vi "Example UDP send MC commands loop.vi"() -> ()   [LabVIEW 2009]
uses:
  UDP Lib/UDP Network Location.ctl
  Remote Control/Motor Command.ctl
  Remote Control/Message Type.ctl
panel:
  in  "Destination Location":T1
  in  "stop":bool
  in  "Turn":i16
  in  "Speed":i16
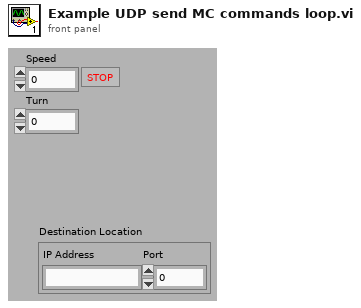
[diagram p1: front panel]
types:
  T1 = typedef "UDP Network Location.ctl" = cluster{"IP Address":string, "Port":u16}
  T2 = typedef "UDP Base.ctl" = cluster{"UDP Session":refnum<k16>, "UDP Socket Params":T3}
  T3 = typedef "UDP Socket Params.ctl" = cluster{"Local Port":u16, "Read Timeout":i32, "Write Timeout":i32}
  T4 = typedef "Message Type.ctl" = enum16{"Motor Command", "Debug Data"}
  T5 = typedef "Motor Command.ctl" = cluster{"Speed":i16, "Turn":i16}
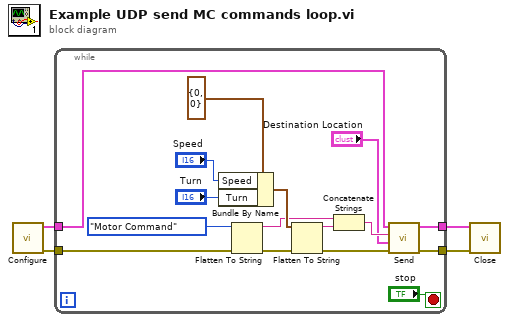
[diagram p0: block diagram]
diagram:
  n1 = call "Configure.vi"() -> ("error out"=w3:errorcluster, "UDP Base out"=w4:T2)  [unwired: 10 in]
  n2 = while {
    tunnel: w4 -> [w7]
    tunnel: w3 -> [w15]
    tunnel: [w9] -> w2
    tunnel: [w8] -> w1
    stop <- "stop" stop-if-true
    n3 = Bundle By Name(cluster=T5 {"Speed"=0, "Turn"=0} ("Motor Command"), "Speed"="Speed", "Turn"="Turn") -> (w14:T5)
    n4 = Flatten To String(anything=Message_Type."Motor Command" ("Message Type"), error in (no error)=w15) -> (data string=w13:string, error out=w6:errorcluster)  [unwired: 2 in, 1 out]
    n5 = Flatten To String(anything=w14, error in (no error)=w6) -> (data string=w12:string, error out=w5:errorcluster)  [unwired: 2 in, 1 out]
    n6 = Concatenate Strings(w13, w12) -> (w11:string)
    n7 = call "Send.vi"("error in (no error)"=w5, "Destination Location"="Destination Location", "Send Data"=w11, "UDP Base in"=w7) -> ("error out"=w8:errorcluster, "UDP Base out"=w9:T2)  [unwired: 5 in, 1 out]
  }
  n8 = call "Close.vi"("error in (no error)"=w1, "Cluster of class private data"=w2) -> ()  [unwired: 9 in, 1 out]
